vi "String Contains.vi"(3 "Regular expression":string="STOP", 4 "Case Sensitive?":bool, 5 "Input String":string) -> (1 "Found?":bool, 2 "Matched String":string)   [LabVIEW 2016]
doc: "This VI finds out if a string contains an expression and returns a true or false boolean."
panel:
  out "after substring":string
  out "before substring":string
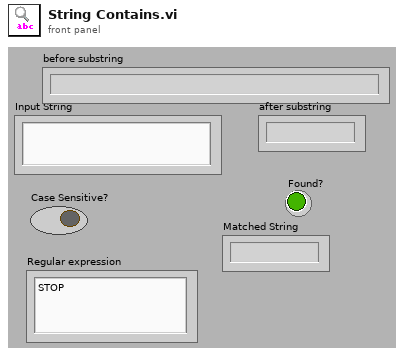
[diagram p1: front panel]
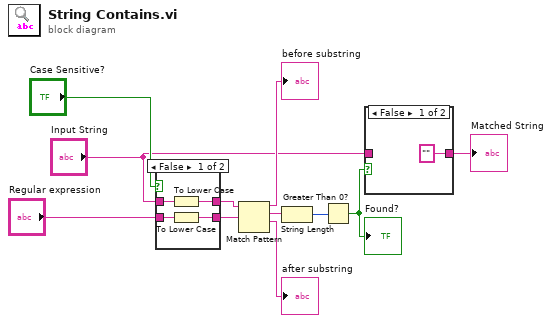
[diagram p0: block diagram]
diagram:
  n1 = case shown="False" "Case Sensitive?" {
    tunnel: "Regular expression" -> [w13 w17]
    tunnel: [w12 w17] -> w7
    tunnel: [w14 w16] -> w6
    tunnel: "Input String" -> [w15 w16]
    frame False {
      n2 = To Lower Case(string=w15) -> (all lower case string=w14:string)
      n3 = To Lower Case(string=w13) -> (all lower case string=w12:string)
    }
    frame True {
    }
  }
  n4 = Match Pattern(string=w6, regular expression=w7) -> (before substring=→"before substring":string, match substring=w10:string, after substring=→"after substring":string)  [unwired: 1 in, 1 out]
  n5 = String Length(string=w10) -> (length=w11:i32)
  n6 = Greater Than 0?(x=w11) -> (x > 0?=w3:bool)
  "Found?" <- w3
  n7 = case shown="False" w3 {
    tunnel: ["" ("Input String") w19] -> w1
    tunnel: "Input String" -> [_ w19]
    frame False {
    }
    frame True {
    }
  }
  "Matched String" <- w1
